vi "WPI_CANTalonSRX_SetOutput.vi"(8 "error in":errorcluster, 9 "Parameter Slot":u8, 10 "Output":dbl, 11 "MotorControlDevRef":T1={"DeviceStatus"={"status"=FALSE, "code"=0, "source"=""}, "Type"=enum."PWM", "PWM"={"PWM Channel"=enum."Invalid", "DeadBand"={"Name"="", "maxPositivePwm"=0, "minPositivePwm"=0, "centerPwm"=0, "maxNegativePwm"=0, "minNegativePwm"=0, "angularRange"=0}}, "CAN"={"Device Number"=0, "SetOutput VI Ref"=variant(enum8{"Percent VBus", "Current", "Speed", "Position", "Voltage"} enum."Percent VBus"), "GetOutput VI Ref"=variant(refnum<k1> refnum), "Enable VI Ref"=variant(dbl 12.0), "Disable VI Ref"=variant(enum8{"Percent VBus", "Speed", "Position", "Slave", "Unchanged / Invalid", "Voltage Compensation", "Current", "Motion Profile"} enum."Percent VBus"), "Data"=variant}, "Invert"=FALSE}) -> (0 "error out":errorcluster, 2 "Motor Output":dbl, 3 "MotorControlDevRef":T1={"DeviceStatus"={"status"=FALSE, "code"=0, "source"=""}, "Type"=enum."PWM", "PWM"={"PWM Channel"=enum."Invalid", "DeadBand"={"Name"="", "maxPositivePwm"=0, "minPositivePwm"=0, "centerPwm"=0, "maxNegativePwm"=0, "minNegativePwm"=0, "angularRange"=0}}, "CAN"={"Device Number"=0, "SetOutput VI Ref"=variant(enum8{"Percent VBus", "Current", "Speed", "Position", "Voltage"} enum."Percent VBus"), "GetOutput VI Ref"=variant(refnum<k1> refnum), "Enable VI Ref"=variant(dbl 12.0), "Disable VI Ref"=variant(enum8{"Percent VBus", "Speed", "Position", "Slave", "Unchanged / Invalid", "Voltage Compensation", "Current", "Motion Profile"} enum."Percent VBus"), "Data"=variant}, "Invert"=FALSE})   [LabVIEW 2016]
doc: "Specifies the output value or set-point for the motor controller.\n\nIf you use a motor controller connected to PWM, the scaled value can range from -1.0 to 1.0.\n\nIf you use a CAN Jaguar, the scale and the units depend on the mode the Jaguar is in. In <B>Percent VBus</B> mode, the range is the same as the PWM interface. In <B>Voltage</B>, <B>Current</B>, <B>Speed</B>, and <B>Position</B> modes, the <B>Output</B> is specified in engineering units (Volts, Amps, Rotations/Minute, and Rotations respectively).\n\nIf you use a CAN Talon SRX, the scale and the units depend on the mode the Talon SRXis in. In <B>Percent VBus</B> mode, the range is the same as the PWM interface. In <B>Speed</B>, and <B>Position</B> modes, the <B>Output</B> is specified in raw sensor units (ticks and ticks / 100 ms respectively).\n\nThis software is licensed. Open the labview\\readme\\WPI Robotics Library Open Source License.txt file for more information."
uses:
  <vilib>/Rock Robotics/WPI/MotorControl/WPI_MotorControlDeviceRef.ctl
  <vilib>/Rock Robotics/WPI/MotorControl/WPI_MotorControlType.ctl
  <vilib>/Rock Robotics/SystemInterfaces/DIO/FPGA_DIOPWMChannel.ctl
  <vilib>/Rock Robotics/WPI/PWM/WPI_PWMDeadband.ctl
  WPI_CANTalonSRX_GlobalOps.ctl
  <vilib>/Rock Robotics/WPI/MotorControl/WPI_MotorControlSafetyCheck.vi
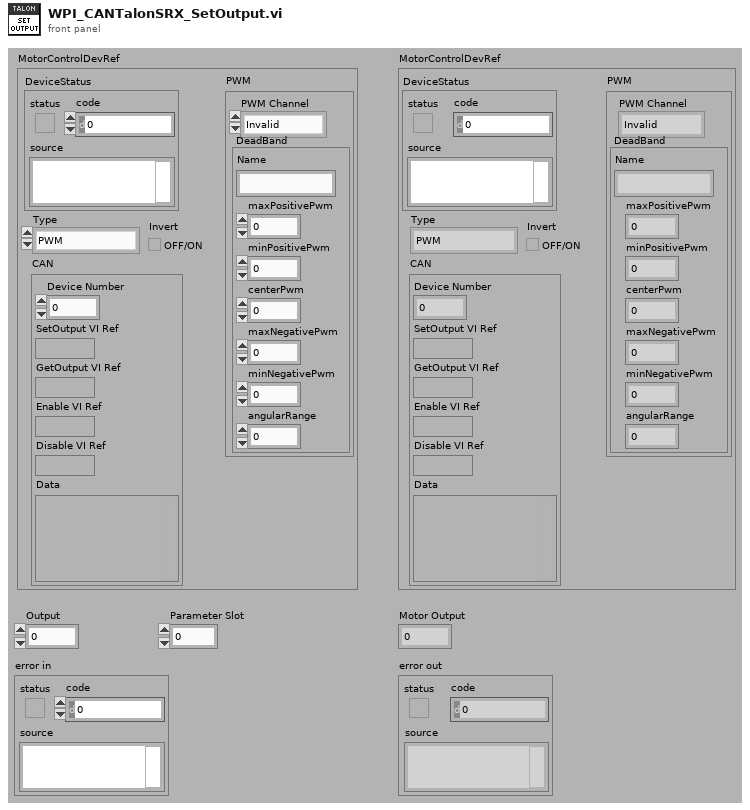
[diagram p1: front panel]
types:
  T1 = typedef "WPI_MotorControlDeviceRef.ctl" = cluster{"DeviceStatus":errorcluster, "Type":T2, "PWM":cluster{"PWM Channel":T3, "DeadBand":T4}, "CAN":cluster{"Device Number":u8, "SetOutput VI Ref":variant, "GetOutput VI Ref":variant, "Enable VI Ref":variant, "Disable VI Ref":variant, "Data":variant}, "Invert":bool}
  T2 = typedef "WPI_MotorControlType.ctl" = enum16{"PWM", "CAN"}
  T3 = typedef "FPGA_DIOPWMChannel.ctl" = enum8{"PWM 0", "PWM 1", "PWM 2", "PWM 3", "PWM 4", "PWM 5", "PWM 6", "PWM 7", "PWM 8", "PWM 9", "PWM MXP 0", "PWM MXP 1", "PWM MXP 2", "PWM MXP 3", "PWM MXP 4", "PWM MXP 5", "PWM MXP 6", "PWM MXP 7", "PWM MXP 8", "PWM MXP 9", "Invalid"}
  T4 = typedef "WPI_PWMDeadband.ctl" = cluster{"Name":string, "maxPositivePwm":i32, "minPositivePwm":i32, "centerPwm":i32, "maxNegativePwm":i32, "minNegativePwm":i32, "angularRange":u16}
  T5 = typedef "WPI_CANTalonSRX_GlobalOps.ctl" = enum16{"Read For Send", "Write After Receive General", "Write After Receive Feedback", "Write After Receive Encoder", "Write After Receive Ain", "Write Error", "Get All", "Set Output", "Set Mode", "Set Master ID", "Set Brake Mode", "Set Reverse Feedback Sensor", "Set Reverse Closed Loop Output", "Set Override Limits", "Set Forward Limit Enabled", "Set Reverse Limit Enabled", "Set Feedback Select", "Set Profile Select", "Set Throttle Ramp Rate", "Disable", "Set Enc Codes Per Rev", "Set Num Pot Turns", "Set Control Frame Rate", "Enable Legacy Control", "Write After Receive Pulse Width", "Set Enable Frame Rate", "Write After Receive Motion Profile", "Set Motion Profile Flow Control", "Set Motion Profile Control Frame Rate", "Set Current Limit Enable"}
  T6 = typedef "WPI_CANTalonSRX_GlobalStatus.ctl" = cluster{"Applied Throttle":dbl, "Module Enabled":bool, "CAN Error":errorcluster, "Closed Loop Error":dbl, "Forward Limit Switch Closed":bool, "Reverse Limit Switch Closed":bool, "Sensor Position":dbl, "Sensor Velocity":dbl, "Current":dbl, "Sticky Fault - Over Temp":bool, "Sticky Fault - Under Voltage":bool, "Sticky Fault - Forward Limit":bool, "Sticky Fault - Reverse Limit":bool, "Sticky Fault - Forward Soft Limit":bool, "Sticky Fault - Reverse Soft Limit":bool, "Brake is Enabled":bool, "Encoder Position":dbl, "Encoder Velocity":dbl, "Encoder Index Count":dbl, "Encoder A Pin State":bool, "Encoder B Pin State":bool, "Encoder Index Pin State":bool, "Analog In":dbl, "Analog In Velocity":dbl, "Temperature (C)":dbl, "Battery Voltage":dbl, "Control 5 Is Supported":bool, "Current Profile Slot Select":dbl, "Pos Div 8":bool, "Vel Div 4":bool, "Pulse Width Position":i32, "Pulse Width Velocity":i32, "Pulse Width Rise To Rise (us)":i32, "Pulse Width Rise To Fall (us)":i32, "Mot Prof Active Is Under Run":bool, "Mot Prof Active Has Under Run":bool, "Mot Prof Active Is Last":bool, "Mot Prof Active Velocity Only":bool, "Mot Prof Active Is Valid":bool, "Mot Prof Buffer Is Full":bool, "Mot Prof Active Profile Slot Select":i32, "Mot Prof NextID":i32, "Mot Prof Count":i32, "Mot Prof Active Velocity":dbl, "Mot Prof Active Position":dbl, "Mot Prof Output Enable":i32}
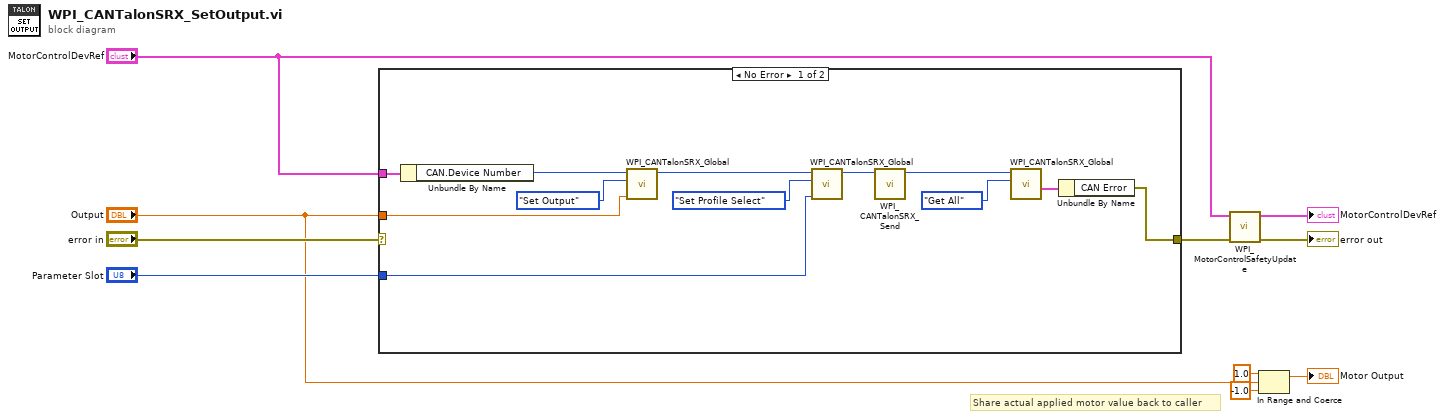
[diagram p0: block diagram]
diagram:
  # "Share actual applied motor value back to caller"
  n1 = case shown="No Error" "error in" {
    selector: "error in" -> [_ w23]
    tunnel: [w22 w23] -> w8
    tunnel: "MotorControlDevRef" -> [w21 _]
    tunnel: "Output" -> [w20 _]
    tunnel: "Parameter Slot" -> [w19 _]
    frame No Error {
      n2 = Unbundle By Name(w21) -> ("CAN.Device Number"=w18:u8)
      n3 = call "WPI_CANTalonSRX_Global.vi"("Set Number"=w20, "Operation"=WPI_CANTalonSRX_GlobalOps."Set Output", "Device ID (0)"=w18) -> ("Device ID Out"=w12:u8)  [unwired: 6 in, 2 out]
      n4 = call "WPI_CANTalonSRX_Global.vi"("Set Number"=w19, "Operation"=WPI_CANTalonSRX_GlobalOps."Set Profile Select", "Device ID (0)"=w12) -> ("Device ID Out"=w11:u8)  [unwired: 6 in, 2 out]
      n5 = call "WPI_CANTalonSRX_Send.vi"("Device ID (0)"=w11) -> ("Device ID Out"=w16:u8)  [unwired: 10 in]
      n6 = call "WPI_CANTalonSRX_Global.vi"("Operation"=WPI_CANTalonSRX_GlobalOps."Get All", "Device ID (0)"=w16) -> ("Get All"=w14:T6)  [unwired: 7 in, 2 out]
      n7 = Unbundle By Name(w14) -> ("CAN Error"=w22:errorcluster)
    }
    frame Error {
    }
  }
  n8 = call <vilib>:"WPI_MotorControlSafetyUpdate.vi"("error in (no error)"=w8, "MotorControlDevRef"="MotorControlDevRef") -> ("error out"=→"error out":errorcluster, "MotorControlDevRef"=→"MotorControlDevRef":T1)  [unwired: 8 out]
  n9 = In Range and Coerce(upper limit=1.0, x="Output", lower limit=-1.0) -> (coerced(x)=→"Motor Output":dbl)  [unwired: 1 out]
